vi "Destroy.vi"(8 "error in (no error)":errorcluster, 11 "reference in":refnum<class "GOOP4_Base.lvclass">) -> (0 "error out":errorcluster, 3 "reference out":refnum<class "GOOP4_Base.lvclass">)   [LabVIEW 2014, in "GOOP4_Base.lvclass"]
uses:
  GOOP4_Base.lvclass
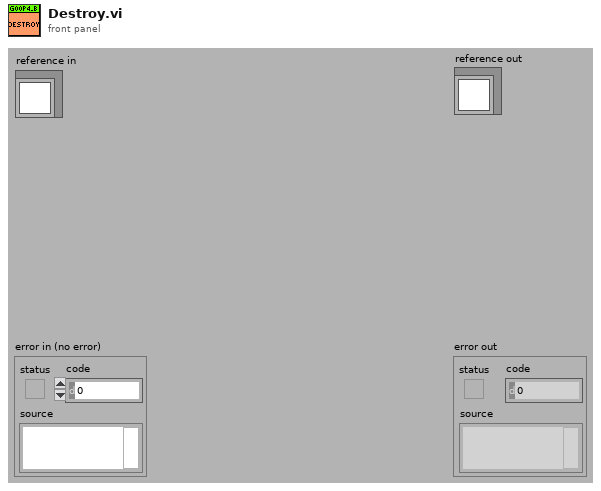
[diagram p1: front panel]
types:
  T1 = typedef "GOOP4_Base.lvclass/ObjectAttributes.ctl" = cluster{"i":i32}
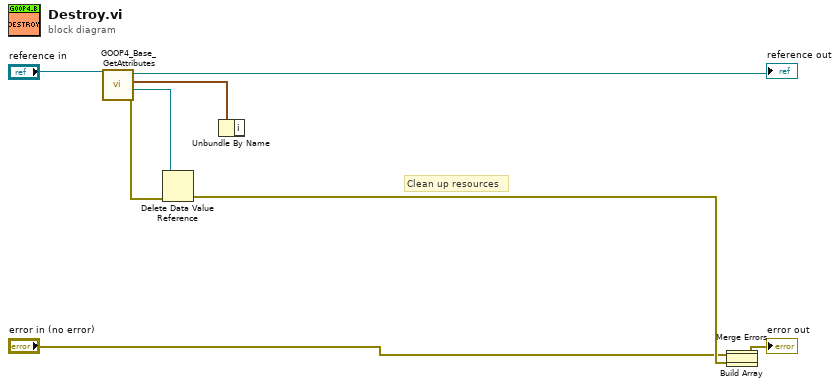
[diagram p0: block diagram]
diagram:
  # "Clean up resources"
  n1 = call "GOOP4_Base_GetAttributes.vi"("reference in"="reference in") -> ("error out"=w6:errorcluster, "DataRef"=w5:refnum<data-value>, "Data"=w4:T1, "reference out"=→"reference out":refnum<class "GOOP4_Base.lvclass">)  [unwired: 7 in]
  n2 = Delete Data Value Reference(data value reference=w5, error in=w6) -> (error out=w3:errorcluster)  [unwired: 1 out]
  n3 = Unbundle By Name(w4) -> ()  [unwired: 1 out]
  n4 = Build Array("error in (no error)", w3) -> (w1:errorcluster[])
  n5 = Merge Errors(w1) -> (→"error out":errorcluster)
